vi "plot radici.vi"(2 "Parte Reale":cluster{"Re1":dbl, "Re2":dbl}, 3 "Coefficienti":cluster{"a":i16, "b":i16, "c":i16}) -> (0 "Asse Y":dbl[](array[numeric]), 1 "Asse X":dbl[](array[numeric]))   [LabVIEW 2021]
panel:
  out "Array":dbl[](array[numeric])
  out "deleted portion":dbl[](array[numeric])
  out "Plot Radici":cluster{"Y":dbl[], "Y":dbl[]}[](graph)
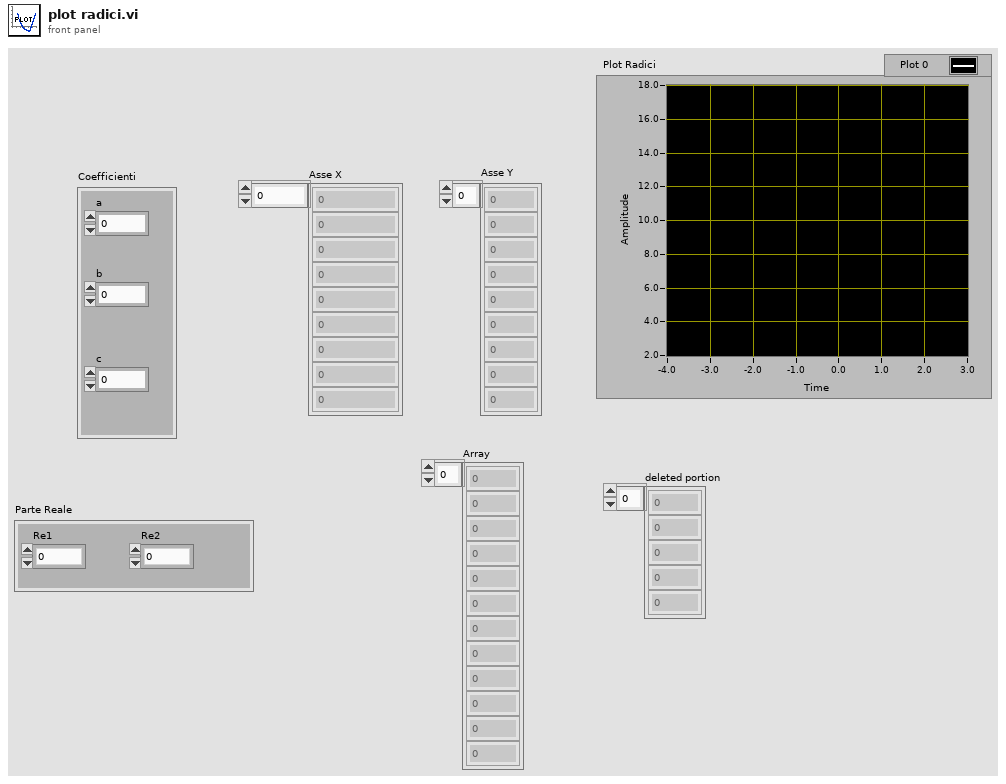
[diagram p1: front panel]
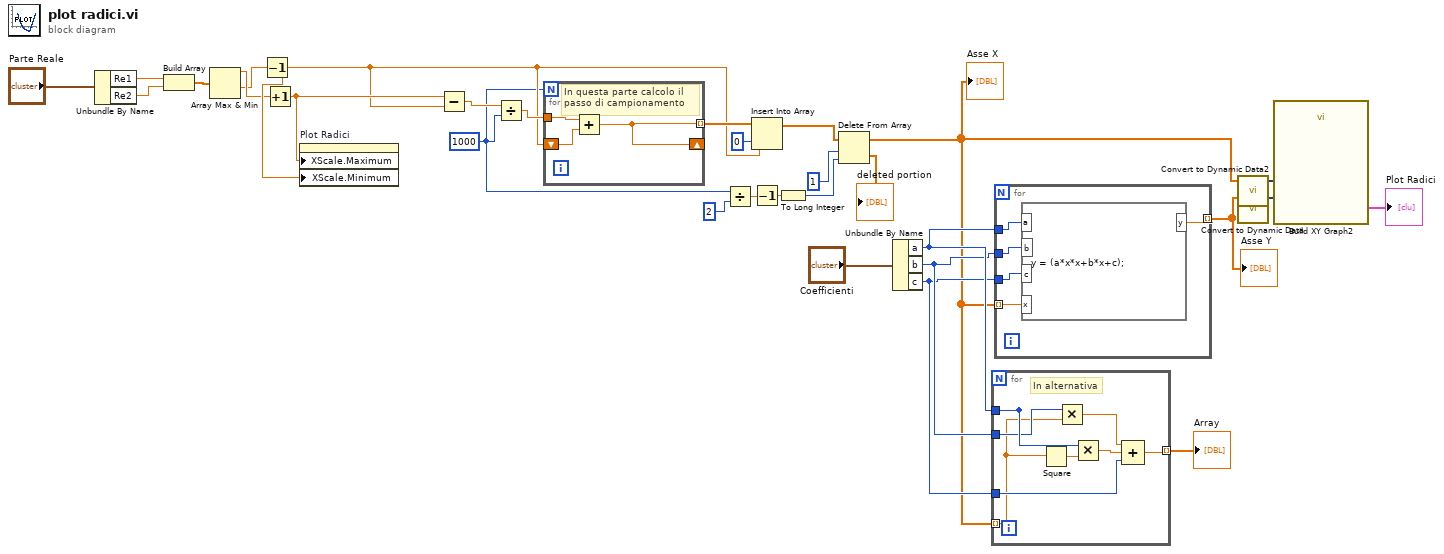
[diagram p0: block diagram]
diagram:
  w15 = 1000
  n1 = Unbundle By Name("Parte Reale") -> ("Re1"=w20:dbl, "Re2"=w19:dbl)
  n2 = Build Array(w20, w19) -> (w18:dbl[])
  n3 = Array Max & Min(array=w18) -> (max value=w17:dbl, min value=w16:dbl)  [unwired: 2 out]
  n4 = Decrement(x=w16) -> (x-1=w22:dbl)
  n5 = Increment(x=w17) -> (x+1=w23:dbl)
  n6 = property on="Plot Radici" class="XYGraph (strict)"("XScale.Maximum"=w23, "XScale.Minimum"=w22) -> ()  [unwired: 2 in, 2 out]
  n7 = Subtract(x=w23, y=w22) -> (x-y=w30:dbl)
  n8 = Divide(x=w30, y=w15) -> (x/y=w29:dbl)
  n9 = for {
    N: w15 -> [_]
    tunnel: w29 -> [w33]
    shift-right: [w31] -> _
    shift-left: w22 -> [w32]
    tunnel: [w31] -> w28 mode=indexing
    # "In questa parte calcolo il\npasso di campionamento"
    n10 = Add(x=w33, y=w32) -> (x+y=w31:dbl)
  }
  n11 = Divide(x=w15, y=2) -> (x/y=w13:dbl)
  n12 = Insert Into Array(array=w28, index=0, new element=w22) -> (w26:dbl[])
  n13 = Decrement(x=w13) -> (x-1=w6:dbl)
  n14 = To Long Integer(number=w6) -> (32bit integer=w12:i32)
  n15 = Delete From Array(array=w26, length=1, index=w12) -> (deleted portion=→"deleted portion":dbl[], array with subset deleted=w5:dbl[])
  "Asse X" <- w5
  n16 = Unbundle By Name("Coefficienti") -> ("a"=w10:i16, "b"=w9:i16, "c"=w8:i16)
  n17 = for {
    tunnel: w5 -> [w37] mode=indexing
    tunnel: [w36] -> w7 mode=indexing
    tunnel: [w40] -> _
    tunnel: w10 -> [w40]
    tunnel: w9 -> [w38]
    tunnel: w8 -> [w39]
    # "In alternativa"
    n18 = Square(x=w37) -> (x^2=w41:dbl)
    n19 = Multiply(x=w38, y=w37) -> (x*y=w35:dbl)
    n20 = Multiply(x=w40, y=w41) -> (x*y=w34:dbl)
    n21 = Compound Arithmetic op=ADD(w35, w34, w39) -> (w36:dbl)
  }
  "Array" <- w7
  n22 = for {
    tunnel: w10 -> [w46]
    tunnel: w9 -> [w45]
    tunnel: w8 -> [w44]
    tunnel: [w43] -> w3 mode=indexing
    tunnel: w5 -> [w42] mode=indexing
    # "Con nodo \"formula\""
    n23 = formula code="y = (a*x*x+b*x+c);"("a"=w46, "b"=w45, "c"=w44, "x"=w42) -> ("y"=w43:dbl)
  }
  "Asse Y" <- w3
  n24 = call "Convert to Dynamic Data2"("Array"=w5) -> ("Dynamic Data Type"=w4:dynamicdata)  [unwired: 3 in]
  n25 = call "Convert to Dynamic Data"("Array"=w3) -> ("Dynamic Data Type"=w2:dynamicdata)  [unwired: 3 in]
  n26 = call "Build XY Graph2"("Y Input"=w2, "X Input"=w4) -> ("XY Graph"=→"Plot Radici":cluster{"X":dbl[], "Y":dbl[]}[])  [unwired: 8 in, 1 out]
